vi "ProdaNG.Example.GetProducts.vi"() -> ()   [LabVIEW 2016]
uses:
  Controls/ProdaNG.Product.ctl
  Controls/ProdaNG.Identification.ctl
panel:
  out "size(s)":i32
  out "Products":T1[](array[typedef])
  out "Prod exist":bool
  out "Result exist":bool
  out "Identification":T2
  out "source":string
  in  "systemName":string="TB_005.01.A_BSV"
  out "ErrCode":i32
  out "error out":errorcluster
  in  "error in (no error)":errorcluster
  in  "wabcoNumber":string="9640050070"
  out "DataBase time":string
  in  "Connection string":string="lcptb/lcptb@PRODA_WPK"
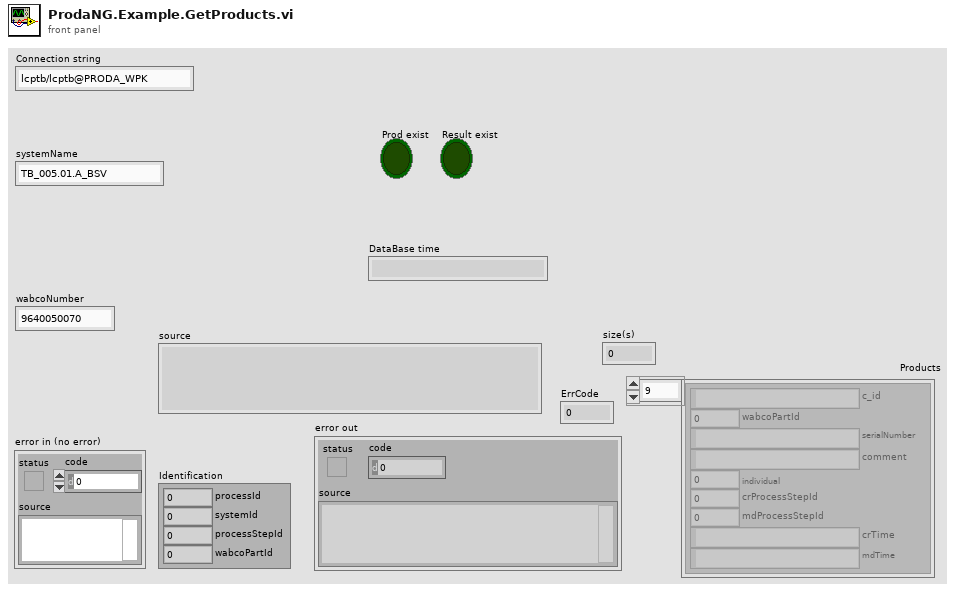
[diagram p1: front panel]
types:
  T1 = typedef "ProdaNG.Product.ctl" = cluster{"c_id":string, "wabcoPartId":i32, "serialNumber":string, "comment":string, "individual":i32, "crProcessStepId":i32, "mdProcessStepId":i32, "crTime":string, "mdTime":string}
  T2 = typedef "ProdaNG.Identification.ctl" = cluster{"processId":i32, "systemId":i32, "processStepId":i32, "wabcoPartId":i32}
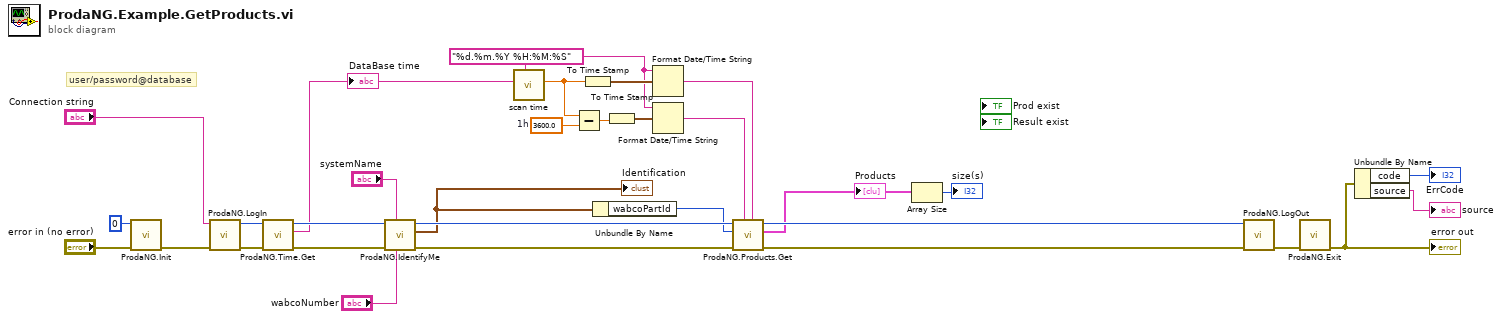
[diagram p0: block diagram]
diagram:
  w7 = 3600.0  # 1h
  w3 = "%d.%m.%Y %H:%M:%S" ("time format string")
  # "user/password@database"
  n1 = call "ProdaNG.Init.vi"("error in (no error)"="error in (no error)", "numContexts (0: unlimited)"=0 ("numContexts")) -> ("error out"=w30:errorcluster)  [unwired: 9 in]
  n2 = call "ProdaNG.LogIn.vi"("error in"=w30, "ConnectionString"="Connection string") -> ("error out"=w26:errorcluster, "dbHandle"=w27:i32)  [unwired: 7 in, 1 out]
  n3 = call "ProdaNG.Time.Get.vi"("error in"=w26, "dbHandleIn"=w27) -> ("error out"=w21:errorcluster, "timeStr"=w9:string, "dbHandle"=w22:i32)  [unwired: 5 in, 1 out]
  "DataBase time" <- w9
  n4 = call "ProdaNG.IdentifyMe.vi"("wabcoNumber"="wabcoNumber", "systemName"="systemName", "error in"=w21, "dbHandleIn"=w22) -> ("error out"=w18:errorcluster, "Identification"=w13:T2, "dbHandle"=w17:i32)  [unwired: 5 in]
  "Identification" <- w13
  n5 = call "scan time.vi"("time format string"=w3, "formatted time string"=w9) -> ("lv time (UTC)"=w8:dbl)  [unwired: 5 in, 4 out]
  n6 = Subtract(x=w8, y=w7) -> (x-y=w6:dbl)
  n7 = To Time Stamp(1:w8) -> (0:w5:timestamp)
  n8 = Unbundle By Name(w13) -> ("wabcoPartId"=w12:i32)
  n9 = To Time Stamp(1:w6) -> (0:w4:timestamp)
  n10 = Format Date/Time String(time format string (%c)=w3, seconds (now)=w5) -> (date/time string=w1:string)  [unwired: 1 in]
  n11 = Format Date/Time String(time format string (%c)=w3, seconds (now)=w4) -> (date/time string=w2:string)  [unwired: 1 in]
  n12 = call "ProdaNG.Products.Get.vi"("Time To"=w1, "Time From"=w2, "error in (no error)"=w18, "wabcoPartId"=w12, "dbHandleIn"=w17) -> ("error out"=w14:errorcluster, "Products"=w11:T1[], "dbHandle"=w15:i32)  [unwired: 3 in, 1 out]
  "Products" <- w11
  n13 = Array Size(array=w11) -> (size(s)=→"size(s)":i32)
  n14 = call "ProdaNG.LogOut.vi"("error in"=w14, "dbHandleIn"=w15) -> ("error out"=w31:errorcluster)  [unwired: 9 in]
  n15 = call "ProdaNG.Exit.vi"("error in (no error)"=w31) -> ("error out"=w23:errorcluster)  [unwired: 10 in]
  "error out" <- w23
  n16 = Unbundle By Name(w23) -> ("code"=→"ErrCode":i32, "source"=→"source":string)
